vi "VNARP-SettingsUpdate.vi"(3 "Error IN":errorcluster caption="entrée d'erreur (pas d'erreur)", 4 "RP VNA SETTINGS IN":T1={"F start"=400000, "F stop"=400000, "Sweep size"=400000, "Decimation"=400000, "F_corr"=400000, "Ph_OUT1"=400000, "Ph_OUT2"=400000, "OUT_Lvl1"=400000, "OUT_Lvl2"=400000, "GPIO"=400000}, 5 "ID de connexion IN":refnum<k5>) -> (0 "Error OUT":errorcluster caption="errreur out", 1 "Freq table":dbl[](array[numeric]), 2 "ID de connexion OUT":refnum<k5>)   [LabVIEW 2021]
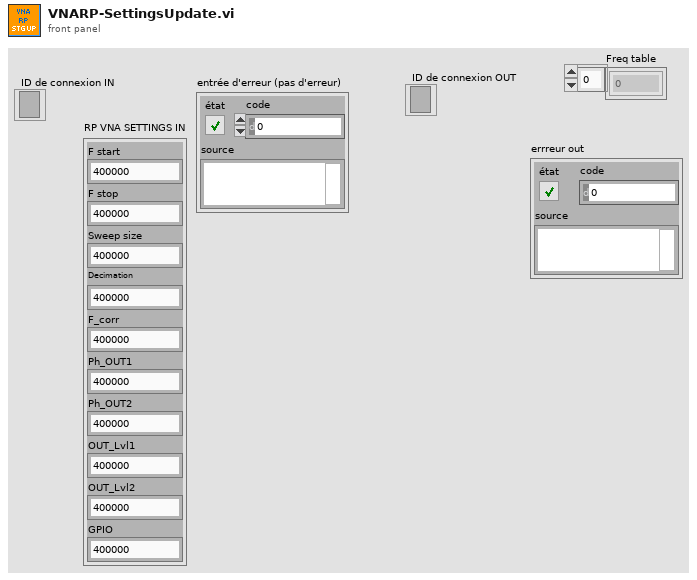
[diagram p1: front panel]
types:
  T1 = cluster{"F start":u32, "F stop":u32, "Sweep size":u32, "Decimation":u32, "F_corr":u32, "Ph_OUT1":u32, "Ph_OUT2":u32, "OUT_Lvl1":u32, "OUT_Lvl2":u32, "GPIO":u32}
  T2 = enum16{"Freq start", "Freq stop", "Sweep size", "Decimation rate", "Freq corr", "Phase output 1", "Phase output 2", "Output level 1", "Output level 2", "GPIO", "SWEEP START"}
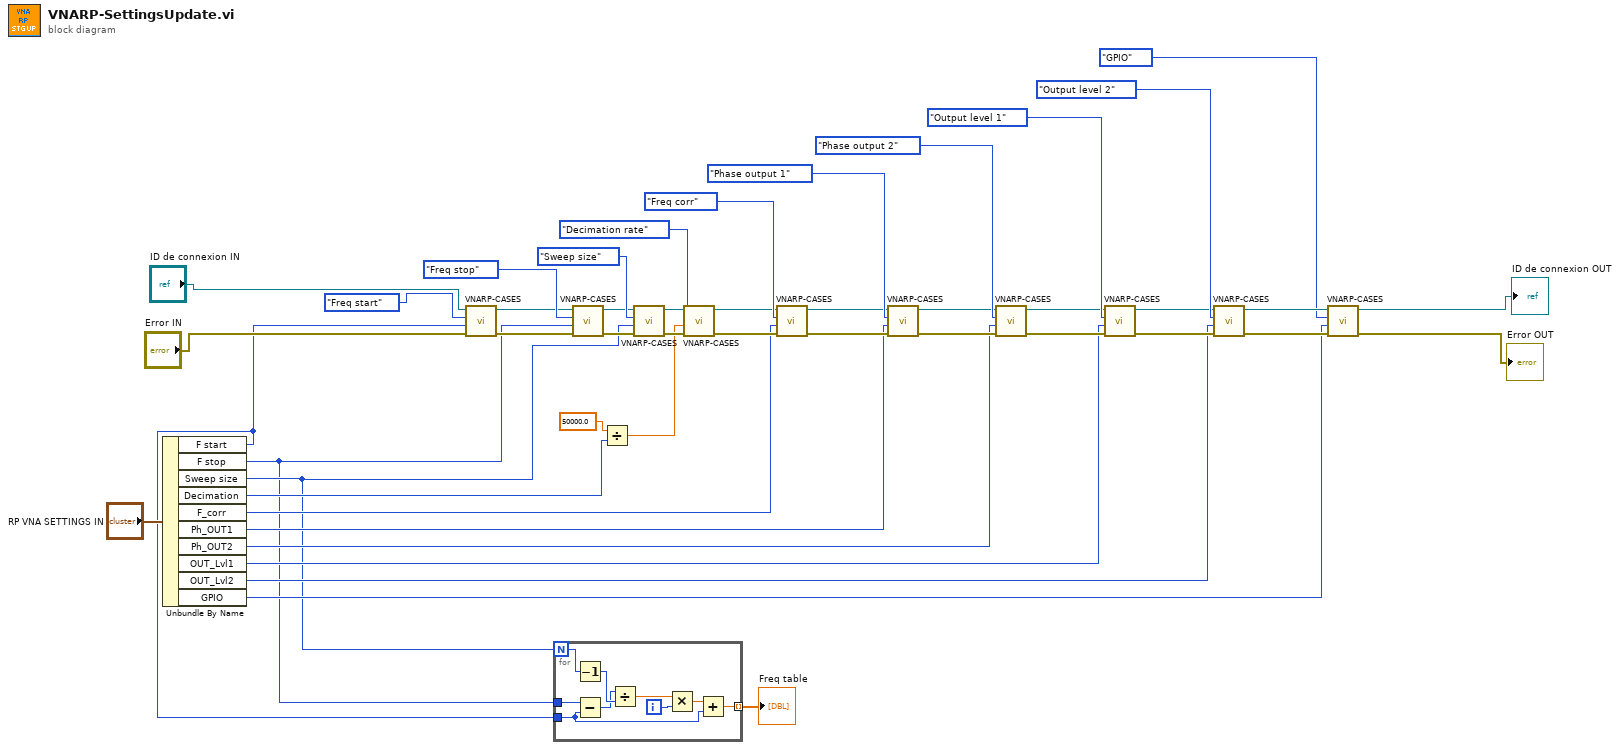
[diagram p0: block diagram]
diagram:
  n1 = Unbundle By Name("RP VNA SETTINGS IN") -> ("F start"=w2:u32, "F stop"=w3:u32, "Sweep size"=w4:u32, "Decimation"=w11:u32, "F_corr"=w10:u32, "Ph_OUT1"=w9:u32, "Ph_OUT2"=w8:u32, "OUT_Lvl1"=w7:u32, "OUT_Lvl2"=w6:u32, "GPIO"=w5:u32)
  n2 = call "VNARP-CASES.vi"("entrée d'erreur (pas d'erreur)"="Error IN", "Setting"=w2, "Énum"=T2."Freq start", "ID de connexion"="ID de connexion IN") -> ("sortie d'erreur"=w44:errorcluster, "ID de connexion en sortie"=w43:refnum<k5>)  [unwired: 3 in]
  n3 = for {
    N: w4 -> [w52]
    tunnel: w3 -> [w54]
    tunnel: w2 -> [w55]
    tunnel: [w48] -> w1 mode=indexing
    i -> [w47]
    n4 = Decrement(x=w52) -> (x-1=w53:i32)
    n5 = Subtract(x=w54, y=w55) -> (x-y=w51:u32)
    n6 = Divide(x=w51, y=w53) -> (x/y=w50:dbl)
    n7 = Multiply(x=w50, y=w47) -> (x*y=w49:dbl)
    n8 = Add(x=w49, y=w55) -> (x+y=w48:dbl)
  }
  "Freq table" <- w1
  n9 = call "VNARP-CASES.vi"("entrée d'erreur (pas d'erreur)"=w44, "Setting"=w3, "Énum"=T2."Freq stop", "ID de connexion"=w43) -> ("sortie d'erreur"=w40:errorcluster, "ID de connexion en sortie"=w41:refnum<k5>)  [unwired: 3 in]
  n10 = Divide(x=50000.0, y=w11) -> (x/y=w17:dbl)
  n11 = call "VNARP-CASES.vi"("entrée d'erreur (pas d'erreur)"=w40, "Setting"=w4, "Énum"=T2."Sweep size", "ID de connexion"=w41) -> ("sortie d'erreur"=w23:errorcluster, "ID de connexion en sortie"=w22:refnum<k5>)  [unwired: 3 in]
  n12 = call "VNARP-CASES.vi"("entrée d'erreur (pas d'erreur)"=w23, "Setting"=w17, "Énum"=T2."Decimation rate", "ID de connexion"=w22) -> ("sortie d'erreur"=w20:errorcluster, "ID de connexion en sortie"=w21:refnum<k5>)  [unwired: 3 in]
  n13 = call "VNARP-CASES.vi"("entrée d'erreur (pas d'erreur)"=w20, "Setting"=w10, "Énum"=T2."Freq corr", "ID de connexion"=w21) -> ("sortie d'erreur"=w37:errorcluster, "ID de connexion en sortie"=w36:refnum<k5>)  [unwired: 3 in]
  n14 = call "VNARP-CASES.vi"("entrée d'erreur (pas d'erreur)"=w37, "Setting"=w9, "Énum"=T2."Phase output 1", "ID de connexion"=w36) -> ("sortie d'erreur"=w30:errorcluster, "ID de connexion en sortie"=w31:refnum<k5>)  [unwired: 3 in]
  n15 = call "VNARP-CASES.vi"("entrée d'erreur (pas d'erreur)"=w30, "Setting"=w8, "Énum"=T2."Phase output 2", "ID de connexion"=w31) -> ("sortie d'erreur"=w33:errorcluster, "ID de connexion en sortie"=w32:refnum<k5>)  [unwired: 3 in]
  n16 = call "VNARP-CASES.vi"("entrée d'erreur (pas d'erreur)"=w33, "Setting"=w7, "Énum"=T2."Output level 1", "ID de connexion"=w32) -> ("sortie d'erreur"=w24:errorcluster, "ID de connexion en sortie"=w25:refnum<k5>)  [unwired: 3 in]
  n17 = call "VNARP-CASES.vi"("entrée d'erreur (pas d'erreur)"=w24, "Setting"=w6, "Énum"=T2."Output level 2", "ID de connexion"=w25) -> ("sortie d'erreur"=w29:errorcluster, "ID de connexion en sortie"=w28:refnum<k5>)  [unwired: 3 in]
  n18 = call "VNARP-CASES.vi"("entrée d'erreur (pas d'erreur)"=w29, "Setting"=w5, "Énum"=T2."GPIO", "ID de connexion"=w28) -> ("sortie d'erreur"=→"Error OUT":errorcluster, "ID de connexion en sortie"=→"ID de connexion OUT":refnum<k5>)  [unwired: 3 in]
